vi "Main.vi"() -> ()   [LabVIEW 2022 SP3]
panel:
  in  "Water Level Chanel":tag
  out "Pump 2 check":bool
  out "Pump 1 check":bool
  in  "Pump 2 Chanel":tag
  in  "Pump 1 Chanel":tag
  in  "stop":bool
  out "Light ON/OFF":bool
  in  "Light Chanel":tag
  out "Boolean":bool
  in  "LDR Input Chanel":tag
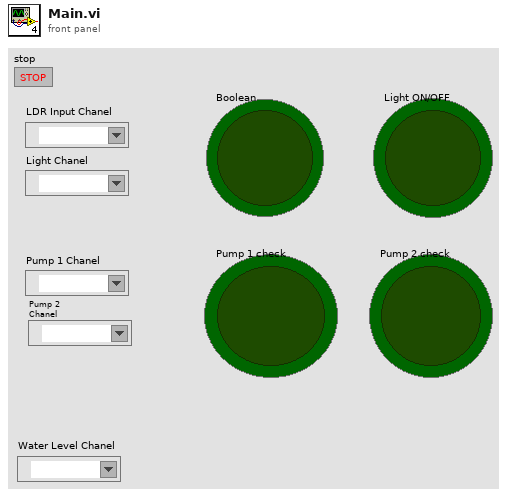
[diagram p1: front panel]
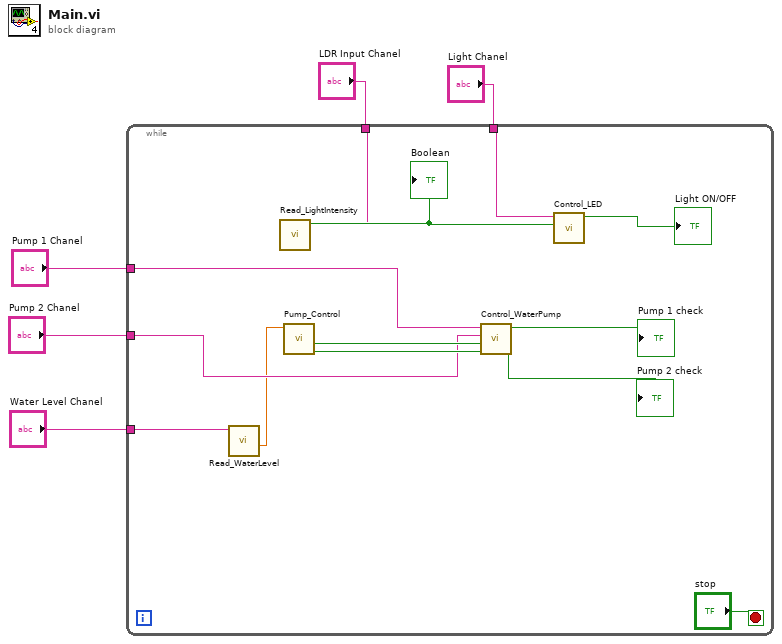
[diagram p0: block diagram]
diagram:
  n1 = while {
    tunnel: "LDR Input Chanel" -> [w15]
    tunnel: "Light Chanel" -> [w14]
    tunnel: "Pump 1 Chanel" -> [w11]
    tunnel: "Pump 2 Chanel" -> [w10]
    tunnel: "Water Level Chanel" -> [w7]
    stop <- "stop" stop-if-true
    n2 = call "Read_WaterLevel.vi"("DAQmx Physical Channel"=w7) -> ("Water Level"=w6:dbl)  [unwired: 8 in, 2 out]
    n3 = call "Read_LightIntensity.vi"("LDR Input"=w15) -> ("Boolean"=w18:bool)  [unwired: 10 in]
    "Boolean" <- w18
    n4 = call "Pump_Control.vi"("Water Level"=w6) -> ("Pump 2 ON"=w12:bool, "Pump 1 ON"=w13:bool)  [unwired: 9 in]
    n5 = call "Control_WaterPump.vi"("Pump 2 Signal"=w12, "Pump 1 Signal"=w13, "Pump 2"=w10, "Pump 1"=w11) -> ("Pump 2 check"=→"Pump 2 check":bool, "Pump 1 check"=→"Pump 1 check":bool)  [unwired: 6 in]
    n6 = call "Control_LED.vi"("Light Signal"=w18, "Light"=w14) -> ("Light ON/OFF"=→"Light ON/OFF":bool)  [unwired: 9 in]
  }
